vi "Set Completed File Attributes.vi"(8 "error in (no error)":errorcluster, 10 "Read-Only":bool, 11 "Data Logging Specification Ref in":T1) -> (0 "error out":errorcluster, 3 "Data Logging Specification Ref out":T1)   [LabVIEW 2020, in "NI_VS Data Logging API.lvlib"]
doc: "Specifies whether log files in the specified data logging specification are set to read-only on completion."
uses:
  <vilib>/NI VeriStand/Execution/DataLogging/NI_VS Data Logging API.lvlib
  <vilib>/NI VeriStand/Execution/DataLogging/DataLoggingSpecification Ref.ctl
  NationalInstruments.VeriStand.ClientAPI
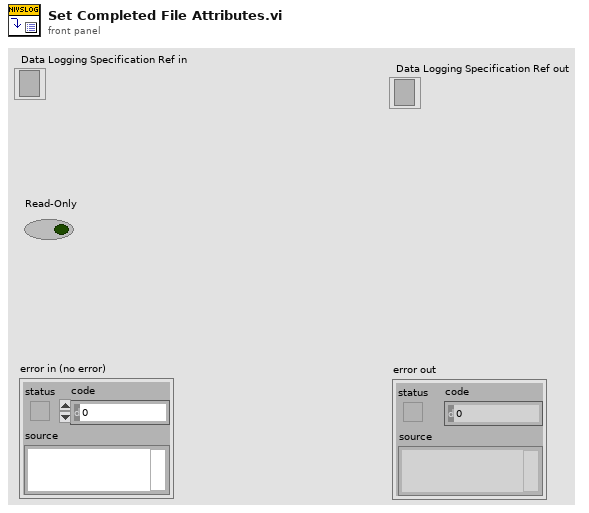
[diagram p1: front panel]
types:
  T1 = typedef "NI_VS Data Logging API.lvlib/DataLoggingSpecification Ref.ctl" = refnum<k24>
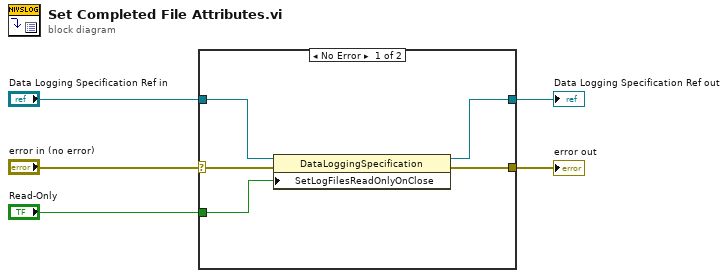
[diagram p0: block diagram]
diagram:
  n1 = case shown="No Error" "error in (no error)" {
    selector: "error in (no error)" -> [w10 w12]
    tunnel: [w9 w12] -> w4
    tunnel: [w6 w11] -> w3
    tunnel: "Data Logging Specification Ref in" -> [w8 w11]
    tunnel: "Read-Only" -> [w7 _]
    frame No Error {
      n2 = property class="DataLoggingSpecification"(reference=w8, error in=w10, "SetLogFilesReadOnlyOnClose"=w7) -> (reference out=w6:T1, error out=w9:errorcluster)
    }
    frame Error {
    }
  }
  "error out" <- w4
  "Data Logging Specification Ref out" <- w3
